vi "DMC CLI VI Analyzer.vi"() -> ()   [LabVIEW 2023]
uses:
  VIA Results Handling/Ranking Thresholds.ctl
  VI Analyzer State.ctl
  <vilib>/Wiresmith Technology/G CLI/CLI Class/CLI.lvclass
  <vilib>/addons/analyzer/_analyzerctrls.llb/VIAnAPI Ref.ctl
  <vilib>/addons/analyzer/_analyzerctrls.llb/VIAnCtl Results.ctl
  <vilib>/addons/analyzer/_analyzerctrls.llb/VIAnCtl ResultsData (index).ctl
  <vilib>/addons/analyzer/_analyzerctrls.llb/VIAnCtl ResultStatus.ctl
  <vilib>/addons/analyzer/_vianresshared.llb/VIAnRes Parsed Results Data (by VI).ctl
  <vilib>/addons/analyzer/_vianresshared.llb/VIAnRes Parsed Results Data (by Test).ctl
  <vilib>/addons/analyzer/_analyzerctrls.llb/VIAnCtl Test Config Data.ctl
  <vilib>/addons/analyzer/_analyzerctrls.llb/VIAnCtl TestRanking.ctl
  <vilib>/addons/analyzer/_analyzerctrls.llb/VIAnCtl Config Control Value.ctl
  <vilib>/Wiresmith Technology/G CLI/Argument Parser/Option Set Class/Option Set.lvclass
  <vilib>/Wiresmith Technology/G CLI/Argument Parser/Option Class/Option Configuration.ctl
  <vilib>/Wiresmith Technology/G CLI/Argument Parser/Option Class/Argument Type.ctl
  07fc47aa-534d-44f0-8168-3e6c46d68514.vi
  <vilib>/addons/analyzer/NI_VIAnalyzerTKVIs.lvlib
  <vilib>/Wiresmith Technology/G CLI/Argument Parser/Option Class/Option.lvclass
  VIA Results Handling/VIA Results Handling.lvlib
panel:
  out "File Paths":path[](array[path])
  out "Custom Parameters":string[](array[string])
  out "Ranking Thresholds":T1={"High"=100.0, "Normal"=90.0, "Low"=80.0}
  out "Per VI Threshold":bool
  out "RSL Report":bool
  out "HTML Report":bool
  out "Excluded Folders":string[](array[string])
  out "Included Folders":string[](array[string])
  in  "Show Results Window?":bool
  out "Results":string
  out "VI in Analysis":string
  out "% Complete":dbl(slide) scale=0.0..100.0
  out "# VIs to Analyze":i32
  out "Report Path":path
  out "Viancfg Path":path
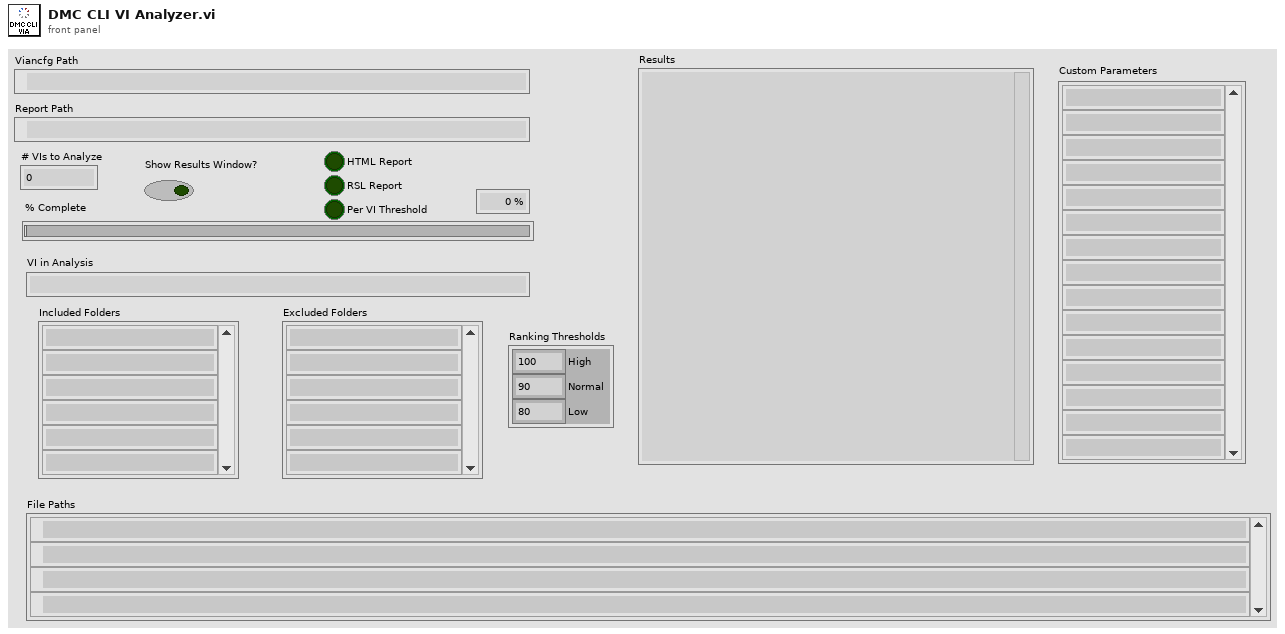
[diagram p1: front panel]
types:
  T1 = typedef "VIA Results Handling.lvlib/Ranking Thresholds.ctl" = cluster{"High":dbl, "Normal":dbl, "Low":dbl}
  T2 = typedef "VIAnAPI Ref.ctl" = refnum<k1>
  T3 = typedef "VIAnCtl Results.ctl" = cluster{"Test Name":string, "Results Data":T4[], "Status":T5, "Exceed Max Fails?":bool}
  T4 = typedef "VIAnCtl ResultsData (index).ctl" = cluster{"Result Message":string, "Ref Index":i32}
  T5 = typedef "VIAnCtl ResultStatus.ctl" = enum16{"Pass", "Fail", "Skipped", "VI not loadable", "Test not loadable", "Test not runnable", "Test error out"}
  T6 = typedef "VIAnRes Parsed Results Data (by VI).ctl" = cluster{"VI Path":path, "Pass":cluster{"row":i32, "column":i32}[], "Fail":cluster{"row":i32, "column":i32}[], "Skipped":cluster{"row":i32, "column":i32}[], "VI not loadable":cluster{"row":i32, "column":i32}[], "Test not loadable":cluster{"row":i32, "column":i32}[], "Test not runnable":cluster{"row":i32, "column":i32}[], "Test error out":cluster{"row":i32, "column":i32}[]}
  T7 = typedef "VIAnRes Parsed Results Data (by Test).ctl" = cluster{"Test Name":string, "Pass":cluster{"VI Path":path, "index":cluster{"row":i32, "column":i32}}[], "Fail":cluster{"VI Path":path, "index":cluster{"row":i32, "column":i32}}[], "Skipped":cluster{"VI Path":path, "index":cluster{"row":i32, "column":i32}}[]}
  T8 = typedef "VIAnCtl Test Config Data.ctl" = cluster{"Test Name":string, "Config Ref":refnum<vi>, "Ref Valid?":bool, "Test Ranking":T9, "Max Failures":u32, "Test Path":path, "Control Values":T10[], "Selected?":bool}
  T9 = typedef "VIAnCtl TestRanking.ctl" = u16
  T10 = typedef "VIAnCtl Config Control Value.ctl" = cluster{"Control Name":string, "Control Value":variant}
  T11 = cluster{"Viancfg Path":path, "Report Directory":path, "CLI":refnum<class "CLI.lvclass">, "VI Analyzer Task":T2, "Analysis Results":cluster{"Raw Results":T3[][], "Parsed Results Data (by VI)":T6[], "Parsed Results Data (by Test)":T7[], "Summary Statistics":cluster{"Passed Tests":i32, "Failed Tests":i32, "Skipped Tests":i32, "VIs not loadable":i32, "Tests not loadable":i32, "Tests not runnable":i32, "Test error out":i32, "Start Time":u32, "Total Time (s)":dbl}, "Test Config Data":T8[]}, "Option Set":refnum<class "Option Set.lvclass">, "Working Directory":path, "Ranking Thresholds":T1, "Included Folders":string[], "Excluded Folders":string[], "HTML Report":bool, "RSL Report":bool, "Per VI Threshold":bool, "Threshold Pass":bool}
  T12 = typedef "VI Analyzer State.ctl" = enum16{"Initialize", "Open viancfg", "Run viancfg", "Include Folders", "Exclude Folders", "Report Threshold", "Report HTML", "Report RSL", "Close", "Help"}
  T13 = enum16{"Viancfg Path", "Report Directory", "Included Folders", "Excluded Folders", "HTML Report", "RSL Report", "Thresholds", "Per VI Threshold"}
  T14 = typedef "Option Parser.lvlib/Option.lvclass/Option Configuration.ctl" = cluster{"Option Type":T15, "Option Labels":string[], "Key":string, "Description":string, "Required":bool, "Default Value":string}
  T15 = typedef "Option Parser.lvlib/Option.lvclass/Argument Type.ctl" = enum16{"flag", "value"}
  T16 = enum16{"open", "replace", "create", "open or create", "replace or create", "replace or create with confirmation"}
  T17 = enum16{"Viancfg Path", "Report Directory", "Included Folders", "Excluded Folders", "HTML Report", "RSL Report", "Thresholds", "Per VI Threshold"}[]
  T18 = cluster{"Raw Results":T3[][], "Parsed Results Data (by VI)":T6[], "Parsed Results Data (by Test)":T7[], "Summary Statistics":cluster{"Passed Tests":i32, "Failed Tests":i32, "Skipped Tests":i32, "VIs not loadable":i32, "Tests not loadable":i32, "Tests not runnable":i32, "Test error out":i32, "Start Time":u32, "Total Time (s)":dbl}, "Test Config Data":T8[]}
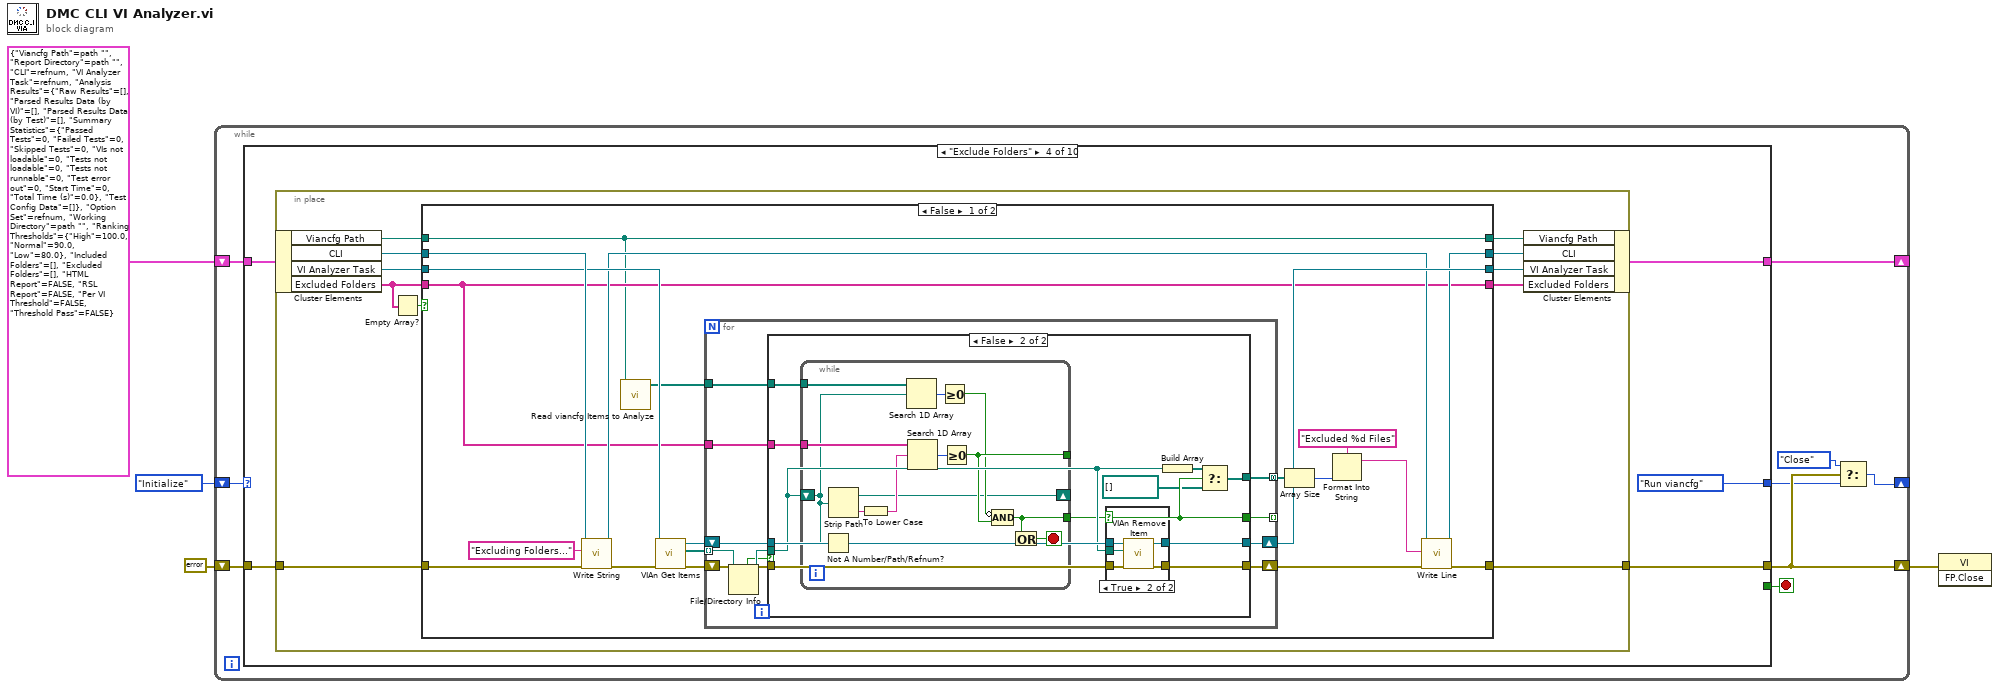
[diagram p0: block diagram]
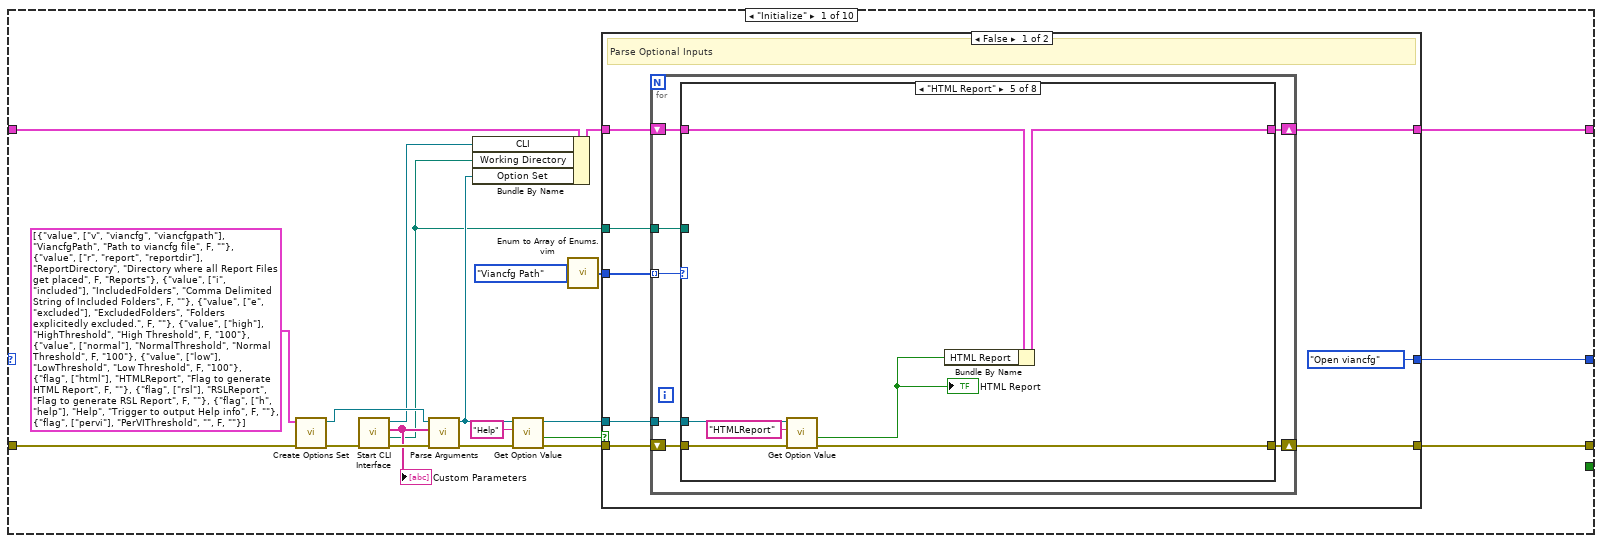
[diagram p2: hidden frame]
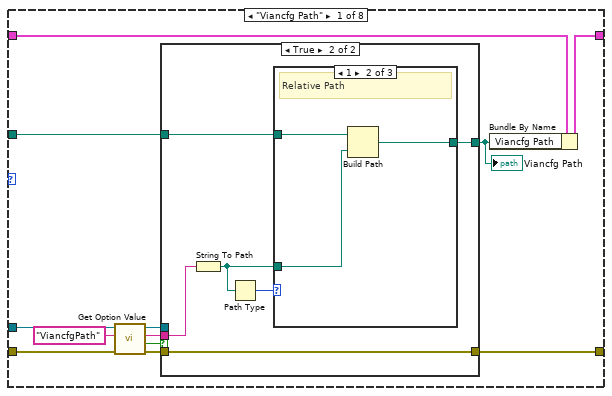
[diagram p3: hidden frame]
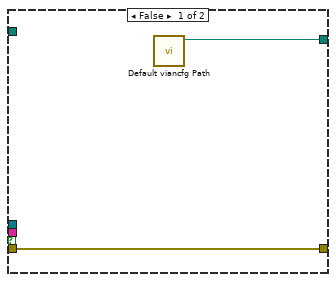
[diagram p4: hidden frame]
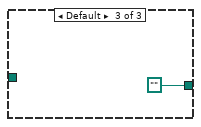
[diagram p6: hidden frame]
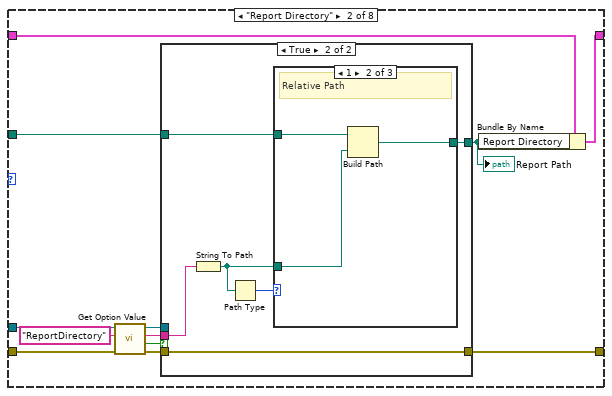
[diagram p7: hidden frame]
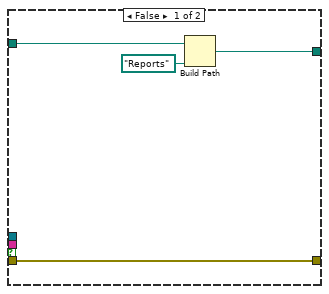
[diagram p8: hidden frame]
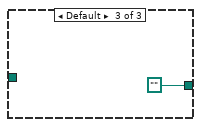
[diagram p10: hidden frame]
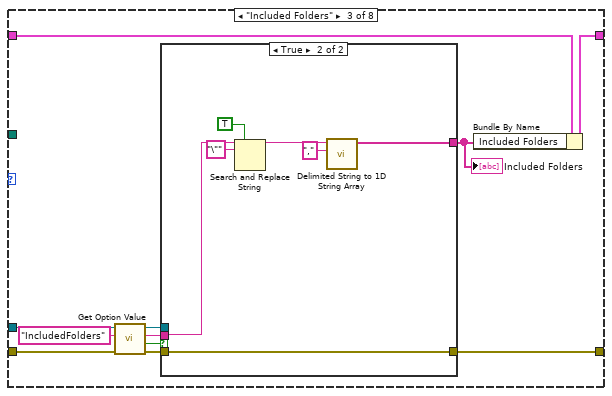
[diagram p11: hidden frame]
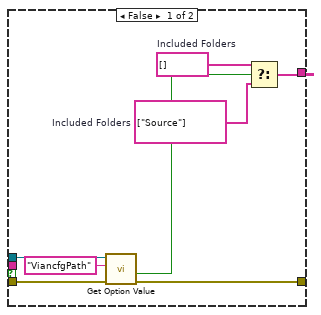
[diagram p12: hidden frame]
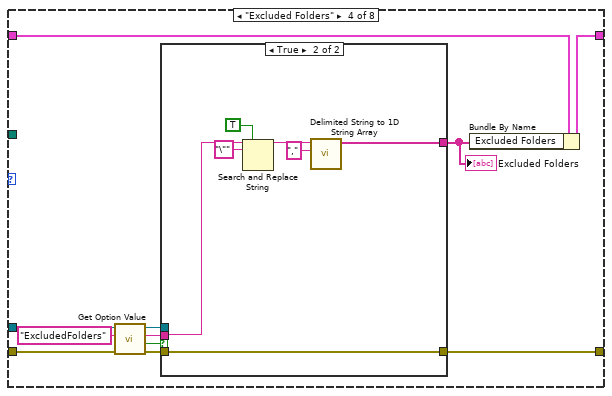
[diagram p13: hidden frame]
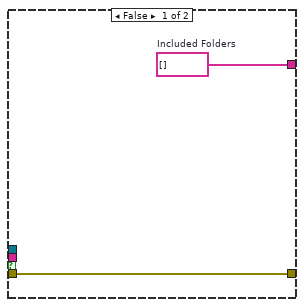
[diagram p14: hidden frame]
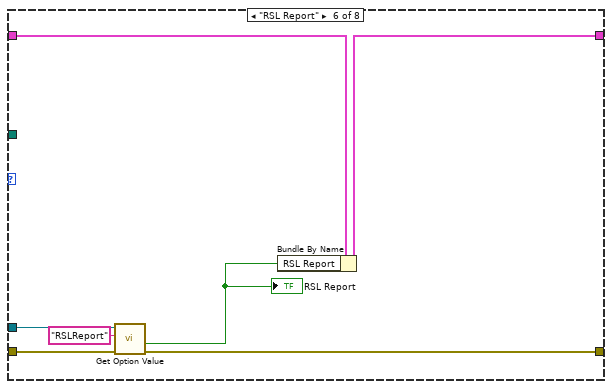
[diagram p15: hidden frame]
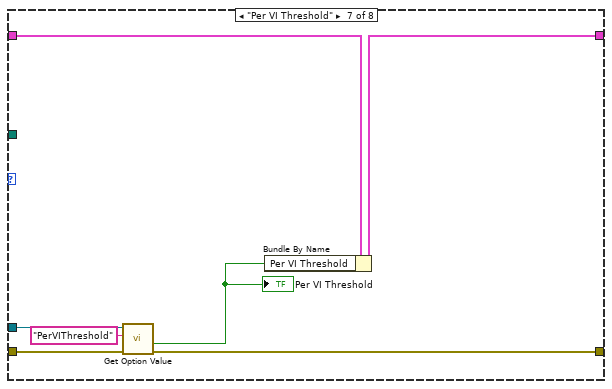
[diagram p16: hidden frame]
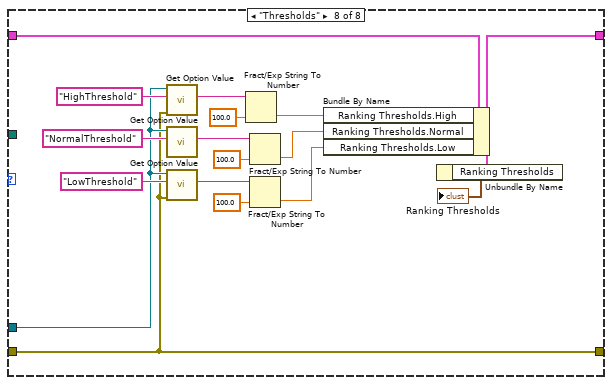
[diagram p17: hidden frame]
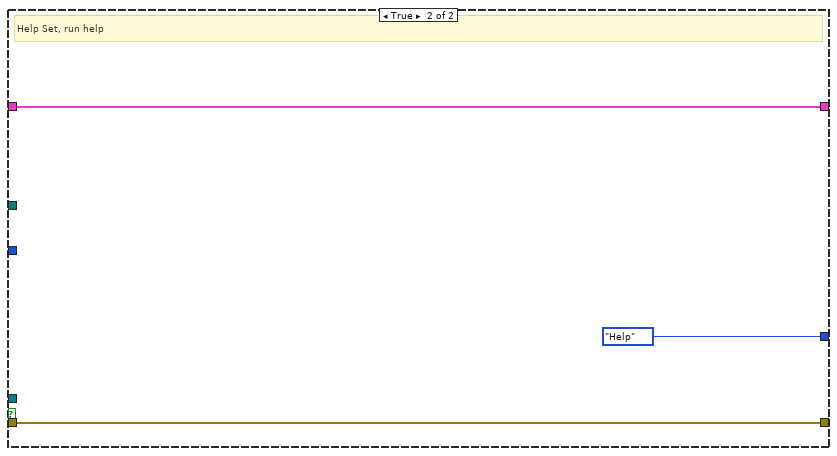
[diagram p18: hidden frame]
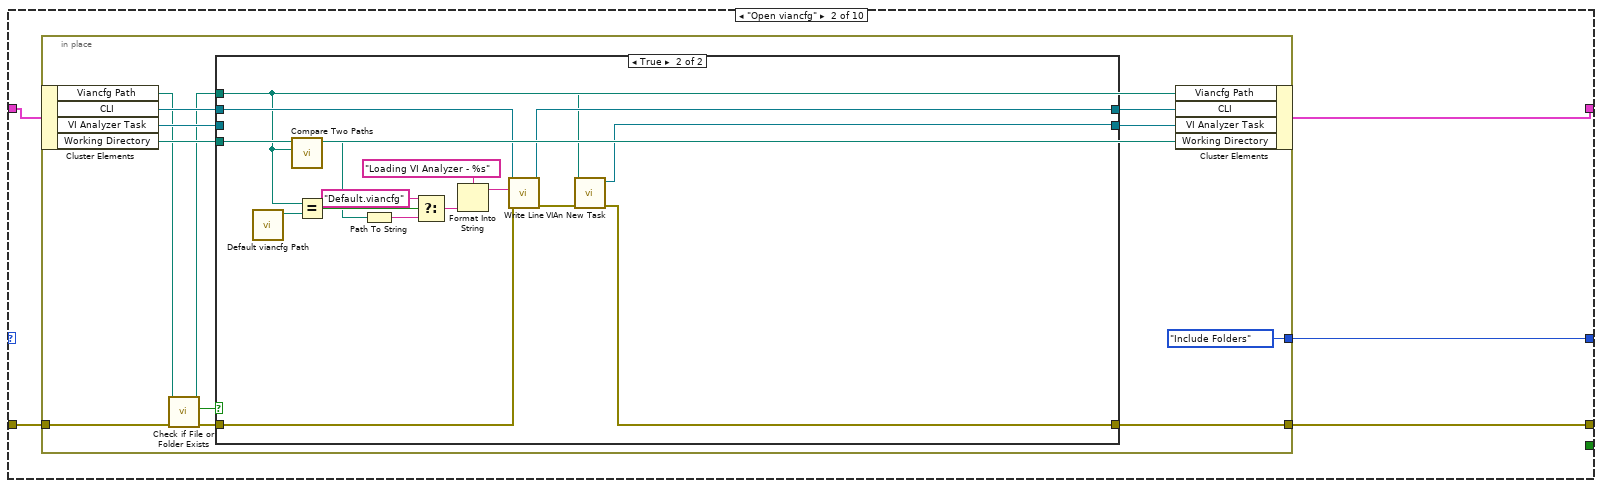
[diagram p19: hidden frame]
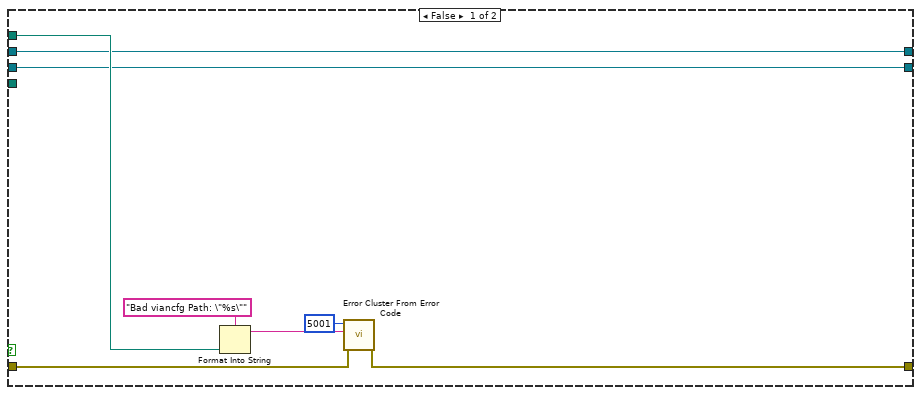
[diagram p20: hidden frame]
diagram:
  n1 = while {
    shift-right: [w6] -> _
    shift-left: VI_Analyzer_State."Initialize" -> [w13]
    shift-right: [w10] -> _
    shift-left: T11 {"Viancfg Path"=path "", "Report Directory"=path "", "CLI"=refnum, "VI Analyzer Task"=refnum, "Analysis Results"={"Raw Results"=[], "Parsed Results Data (by VI)"=[], "Parsed Results Data (by Test)"=[], "Summary Statistics"={"Passed Tests"=0, "Failed Tests"=0, "Skipped Tests"=0, "VIs not loadable"=0, "Tests not loadable"=0, "Tests not runnable"=0, "Test error out"=0, "Start Time"=0, "Total Time (s)"=0.0}, "Test Config Data"=[]}, "Option Set"=refnum, "Working Directory"=path "", "Ranking Thresholds"={"High"=100.0, "Normal"=90.0, "Low"=80.0}, "Included Folders"=[], "Excluded Folders"=[], "HTML Report"=FALSE, "RSL Report"=FALSE, "Per VI Threshold"=FALSE, "Threshold Pass"=FALSE} -> [w12]
    shift-right: [w9] -> w1
    shift-left: errorcluster {"status"=FALSE, "code"=0, "source"=""} ("error out") -> [w11]
    stop <- w5 stop-if-true
    n2 = case shown="\"Exclude Folders\"" w13 {
      tunnel: w12 -> [w34 w193 w234 w322 w438 w506 w540 w573 w619 w621]
      tunnel: w11 -> [w29 w190 w231 w319 w436 w509 w543 w576 w618 w623]
      tunnel: [w14 w192 w233 w321 w437 w510 w544 w577 w619 w620] -> w10
      tunnel: [w18 w191 w232 w320 w435 w508 w542 w575 w615 w622] -> w9
      tunnel: [w33 w189 VI_Analyzer_State."Exclude Folders" VI_Analyzer_State."Run viancfg" w434 w507 w541 w574 VI_Analyzer_State."Close" VI_Analyzer_State."Close"] -> w7
      tunnel: [_ _ _ _ _ _ _ _ TRUE _] -> w5
      frame "Initialize" {
        n3 = call <vilib>:"Create Options Set.vi"("error in (no error)"=w29, "Options"=T14[] [{"Option Type"=enum."value", "Option Labels"=["v", "viancfg", "viancfgpath"], "Key"="ViancfgPath", "Description"="Path to viancfg file", "Required"=FALSE, "Default Value"=""}, {"Option Type"=enum."value", "Option Labels"=["r", "report", "reportdir"], "Key"="ReportDirectory", "Description"="Directory where all Report Files get placed", "Required"=FALSE, "Default Value"="Reports"}, {"Option Type"=enum."value", "Option Labels"=["i", "included"], "Key"="IncludedFolders", "Description"="Comma Delimited String of Included Folders", "Required"=FALSE, "Default Value"=""}, {"Option Type"=enum."value", "Option Labels"=["e", "excluded"], "Key"="ExcludedFolders", "Description"="Folders explicitedly excluded.", "Required"=FALSE, "Default Value"=""}, {"Option Type"=enum."value", "Option Labels"=["high"], "Key"="HighThreshold", "Description"="High Threshold", "Required"=FALSE, "Default Value"="100"}, {"Option Type"=enum."value", "Option Labels"=["normal"], "Key"="NormalThreshold", "Description"="Normal Threshold", "Required"=FALSE, "Default Value"="100"}, {"Option Type"=enum."value", "Option Labels"=["low"], "Key"="LowThreshold", "Description"="Low Threshold", "Required"=FALSE, "Default Value"="100"}, {"Option Type"=enum."flag", "Option Labels"=["html"], "Key"="HTMLReport", "Description"="Flag to generate HTML Report", "Required"=FALSE, "Default Value"=""}, {"Option Type"=enum."flag", "Option Labels"=["rsl"], "Key"="RSLReport", "Description"="Flag to generate RSL Report", "Required"=FALSE, "Default Value"=""}, {"Option Type"=enum."flag", "Option Labels"=["h", "help"], "Key"="Help", "Description"="Trigger to output Help info", "Required"=FALSE, "Default Value"=""}, {"Option Type"=enum."flag", "Option Labels"=["pervi"], "Key"="PerVIThreshold", "Description"="", "Required"=FALSE, "Default Value"=""}]) -> ("error out"=w30:errorcluster, "Option Set out"=w28:refnum<class "Option Set.lvclass">)  [unwired: 8 in]
        n4 = call <vilib>:"Start CLI Interface.vi"("error in (no error)"=w30) -> ("error out"=w32:errorcluster, "Working Directory"=w15:path, "Custom Parameters"=w27:string[], "CLI out"=w23:refnum<class "CLI.lvclass">)  [unwired: 7 in]
        "Custom Parameters" <- w27
        n5 = call <vilib>:"Parse Arguments.vi"("error in (no error)"=w32, "Arguments"=w27, "Option Set in"=w28) -> ("error out"=w25:errorcluster, "Option Set out"=w22:refnum<class "Option Set.lvclass">)  [unwired: 5 in, 2 out]
        n6 = Bundle By Name(cluster=w34, "CLI"=w23, "Working Directory"=w15, "Option Set"=w22) -> (w24:T11)
        n7 = call <vilib>:"Get Option Value.vi"("error in (no error)"=w25, "Option Key"="Help", "Option Set in"=w22) -> ("error out"=w20:errorcluster, "Set"=w21:bool, "Option Set out"=w19:refnum<class "Option Set.lvclass">)  [unwired: 5 in, 1 out]
        n8 = call "Enum to Array of Enums.vim"("enum"=T13."Viancfg Path") -> ("array of enums"=w16:T17)
        n9 = case shown="False" w21 {
          tunnel: [w38 w187] -> w14
          tunnel: [VI_Analyzer_State."Open viancfg" VI_Analyzer_State."Help"] -> w33
          tunnel: w24 -> [w40 w187]
          tunnel: w20 -> [w41 w186]
          tunnel: w19 -> [w42 _]
          tunnel: [w36 w186] -> w18
          tunnel: w16 -> [w39 _]
          tunnel: w15 -> [w37 _]
          frame False {
            # "Parse Optional Inputs"
            n10 = for {
              tunnel: w42 -> [w49]
              shift-right: [w46] -> w38
              shift-left: w40 -> [w45]
              tunnel: w39 -> [w47] mode=indexing
              tunnel: w37 -> [w44]
              shift-right: [w43] -> w36
              shift-left: w41 -> [w48]
              n11 = case shown="\"HTML Report\"" w47 {
                tunnel: w49 -> [w61 w86 w112 w138 w154 w161 w168 w178]
                tunnel: w48 -> [w60 w85 w111 w137 w153 w160 w167 w177]
                tunnel: [w52 w77 w103 w129 w149 w156 w163 w170] -> w46
                tunnel: w45 -> [w54 w79 w105 w131 w151 w158 w165 w184]
                tunnel: w44 -> [w51 w76 _ _ _ _ _ _]
                tunnel: [w53 w78 w104 w130 w150 w157 w164 w177] -> w43
                frame "Viancfg Path" {
                  n12 = call <vilib>:"Get Option Value.vi"("error in (no error)"=w60, "Option Key"="ViancfgPath", "Option Set in"=w61) -> ("error out"=w58:errorcluster, "Set"=w57:bool, "Value"=w55:string, "Option Set out"=w56:refnum<class "Option Set.lvclass">)  [unwired: 5 in]
                  n13 = case shown="True" w57 {
                    tunnel: w58 -> [w63 w68]
                    tunnel: w56 -> [_ _]
                    tunnel: w55 -> [_ w69]
                    tunnel: [w63 w68] -> w53
                    tunnel: [w62 w65] -> w50
                    tunnel: w51 -> [_ w64]
                    frame False {
                      n14 = call "Default viancfg Path.vi"() -> ("Default.viancfg Path"=w62:path)  [unwired: 11 in]
                    }
                    frame True {
                      n15 = String To Path(string=w69) -> (path=w66:path)
                      n16 = Path Type(1:w66) -> (0:w67:i16)
                      n17 = case shown="1" w67 {
                        tunnel: w66 -> [w70 w72 _]
                        tunnel: [w70 w71 path ""] -> w65
                        tunnel: w64 -> [_ w73 _]
                        frame 0 {
                          # "Absolute Path"
                        }
                        frame 1 {
                          # "Relative Path"
                          n18 = Build Path(base path=w73, name or relative path=w72) -> (appended path=w71:path)
                        }
                        frame Default {
                        }
                      }
                    }
                  }
                  "Viancfg Path" <- w50
                  n19 = Bundle By Name(cluster=w54, "Viancfg Path"=w50) -> (w52:T11)
                }
                frame "Report Directory" {
                  n20 = call <vilib>:"Get Option Value.vi"("error in (no error)"=w85, "Option Key"="ReportDirectory", "Option Set in"=w86) -> ("error out"=w83:errorcluster, "Set"=w82:bool, "Value"=w80:string, "Option Set out"=w81:refnum<class "Option Set.lvclass">)  [unwired: 5 in]
                  n21 = case shown="True" w82 {
                    tunnel: w83 -> [w89 w95]
                    tunnel: w81 -> [_ _]
                    tunnel: w80 -> [_ w96]
                    tunnel: [w89 w95] -> w78
                    tunnel: [w88 w92] -> w75
                    tunnel: w76 -> [w87 w91]
                    frame False {
                      n22 = Build Path(base path=w87, name or relative path=path "Reports") -> (appended path=w88:path)
                    }
                    frame True {
                      n23 = String To Path(string=w96) -> (path=w93:path)
                      n24 = Path Type(1:w93) -> (0:w94:i16)
                      n25 = case shown="1" w94 {
                        tunnel: w93 -> [w97 w99 _]
                        tunnel: [w97 w98 path ""] -> w92
                        tunnel: w91 -> [_ w100 _]
                        frame 0 {
                          # "Absolute Path"
                        }
                        frame 1 {
                          # "Relative Path"
                          n26 = Build Path(base path=w100, name or relative path=w99) -> (appended path=w98:path)
                        }
                        frame Default {
                        }
                      }
                    }
                  }
                  "Report Path" <- w75
                  n27 = Bundle By Name(cluster=w79, "Report Directory"=w75) -> (w77:T11)
                }
                frame "Included Folders" {
                  n28 = call <vilib>:"Get Option Value.vi"("error in (no error)"=w111, "Option Key"="IncludedFolders", "Option Set in"=w112) -> ("error out"=w109:errorcluster, "Set"=w108:bool, "Value"=w106:string, "Option Set out"=w107:refnum<class "Option Set.lvclass">)  [unwired: 5 in]
                  n29 = case shown="True" w108 {
                    tunnel: w109 -> [w118 w127]
                    tunnel: w107 -> [w119 _]
                    tunnel: w106 -> [_ w122]
                    tunnel: [w117 w127] -> w104
                    tunnel: [w113 w126] -> w102
                    frame False {
                      w114 = string[] ["Source"]  # Included Folders
                      w115 = string[] []  # Included Folders
                      n30 = call <vilib>:"Get Option Value.vi"("error in (no error)"=w118, "Option Key"="ViancfgPath", "Option Set in"=w119) -> ("error out"=w117:errorcluster, "Set"=w116:bool)  [unwired: 5 in, 2 out]
                      n31 = Select(t=w115, s=w116, f=w114) -> (s? t:f=w113:string[])
                    }
                    frame True {
                      n32 = Search and Replace String(replace all?=TRUE ("replace all? (F)"), input string=w122, search string="\"") -> (result string=w123:string)  [unwired: 5 in, 3 out]
                      n33 = call <vilib>:"Delimited String to 1D String Array.vi"("delimiter"=",", "delimited string"=w123) -> ("string array"=w126:string[])  [unwired: 9 in]
                    }
                  }
                  "Included Folders" <- w102
                  n34 = Bundle By Name(cluster=w105, "Included Folders"=w102) -> (w103:T11)
                }
                frame "Excluded Folders" {
                  n35 = call <vilib>:"Get Option Value.vi"("error in (no error)"=w137, "Option Key"="ExcludedFolders", "Option Set in"=w138) -> ("error out"=w135:errorcluster, "Set"=w134:bool, "Value"=w132:string, "Option Set out"=w133:refnum<class "Option Set.lvclass">)  [unwired: 5 in]
                  n36 = case shown="True" w134 {
                    tunnel: w135 -> [w140 w147]
                    tunnel: w133 -> [_ _]
                    tunnel: w132 -> [_ w141]
                    tunnel: [w140 w147] -> w130
                    tunnel: [w139 w146] -> w128
                    frame False {
                      w139 = string[] []  # Included Folders
                    }
                    frame True {
                      n37 = Search and Replace String(replace all?=TRUE ("replace all? (F)"), input string=w141, search string="\"") -> (result string=w142:string)  [unwired: 5 in, 3 out]
                      n38 = call <vilib>:"Delimited String to 1D String Array.vi"("delimiter"=",", "delimited string"=w142) -> ("string array"=w146:string[])  [unwired: 9 in]
                    }
                  }
                  "Excluded Folders" <- w128
                  n39 = Bundle By Name(cluster=w131, "Excluded Folders"=w128) -> (w129:T11)
                }
                frame "HTML Report" {
                  n40 = call <vilib>:"Get Option Value.vi"("error in (no error)"=w153, "Option Key"="HTMLReport", "Option Set in"=w154) -> ("error out"=w150:errorcluster, "Set"=w148:bool)  [unwired: 5 in, 2 out]
                  "HTML Report" <- w148
                  n41 = Bundle By Name(cluster=w151, "HTML Report"=w148) -> (w149:T11)
                }
                frame "RSL Report" {
                  n42 = call <vilib>:"Get Option Value.vi"("error in (no error)"=w160, "Option Key"="RSLReport", "Option Set in"=w161) -> ("error out"=w157:errorcluster, "Set"=w155:bool)  [unwired: 5 in, 2 out]
                  "RSL Report" <- w155
                  n43 = Bundle By Name(cluster=w158, "RSL Report"=w155) -> (w156:T11)
                }
                frame "Per VI Threshold" {
                  n44 = call <vilib>:"Get Option Value.vi"("error in (no error)"=w167, "Option Key"="PerVIThreshold", "Option Set in"=w168) -> ("error out"=w164:errorcluster, "Set"=w162:bool)  [unwired: 5 in, 2 out]
                  "Per VI Threshold" <- w162
                  n45 = Bundle By Name(cluster=w165, "Per VI Threshold"=w162) -> (w163:T11)
                }
                frame "Thresholds" {
                  n46 = call <vilib>:"Get Option Value.vi"("error in (no error)"=w177, "Option Key"="HighThreshold", "Option Set in"=w178) -> ("Value"=w183:string)  [unwired: 5 in, 3 out]
                  n47 = call <vilib>:"Get Option Value.vi"("Option Key"="NormalThreshold", "Option Set in"=w178) -> ("Value"=w175:string)  [unwired: 6 in, 3 out]
                  n48 = call <vilib>:"Get Option Value.vi"("error in (no error)"=w177, "Option Key"="LowThreshold", "Option Set in"=w178) -> ("Value"=w172:string)  [unwired: 5 in, 3 out]
                  n49 = Fract/Exp String To Number(string=w183, default (0 dbl)=100.0 ("default (0 DBL)")) -> (number=w182:dbl)  [unwired: 2 in, 1 out]
                  n50 = Fract/Exp String To Number(string=w175, default (0 dbl)=100.0 ("default (0 DBL)")) -> (number=w174:dbl)  [unwired: 2 in, 1 out]
                  n51 = Fract/Exp String To Number(string=w172, default (0 dbl)=100.0 ("default (0 DBL)")) -> (number=w171:dbl)  [unwired: 2 in, 1 out]
                  n52 = Bundle By Name(cluster=w184, "Ranking Thresholds.High"=w182, "Ranking Thresholds.Normal"=w174, "Ranking Thresholds.Low"=w171) -> (w170:T11)
                  n53 = Unbundle By Name(w170) -> ("Ranking Thresholds"=→"Ranking Thresholds":T1)
                }
              }
            }
          }
          frame True {
            # "Help Set, run help"
          }
        }
      }
      frame "Open viancfg" {
        n54 = in-place {
          in-place-border: [w203] -> w191
          in-place-border: w190 -> [w194]
          in-place-border: [VI_Analyzer_State."Include Folders"] -> w189
          n55 = in-place-cluster #1(w193) -> ("Viancfg Path"=w198:path, "CLI"=w205:refnum<class "CLI.lvclass">, "VI Analyzer Task"=w202:T2, "Working Directory"=w199:path)
          n56 = call <vilib>:"Check if File or Folder Exists.vi"("error in (no error)"=w194, "path"=w198) -> ("error out"=w195:errorcluster, "file or folder exists?"=w196:bool, "dup path"=w197:path)  [unwired: 7 in]
          n57 = case shown="True" w196 {
            tunnel: w205 -> [w211 w228]
            tunnel: [w211 w225] -> w204
            tunnel: [w208 w224] -> w203
            tunnel: w195 -> [w209 w227]
            tunnel: w197 -> [w212 w219]
            tunnel: w202 -> [w206 _]
            tunnel: [w206 w226] -> w200
            tunnel: w199 -> [_ w223]
            frame False {
              n58 = Format Into String(format string="Bad viancfg Path: \"%s\"", w212) -> (resulting string=w210:string)  [unwired: 2 in, 1 out]
              n59 = call <vilib>:"Error Cluster From Error Code.vi"("error in (no error)"=w209, "error message (\"\")"=w210, "error code (0)"=5001) -> ("error out"=w208:errorcluster)  [unwired: 6 in]
            }
            frame True {
              n60 = call "Default viancfg Path.vi"() -> ("Default.viancfg Path"=w220:path)  [unwired: 11 in]
              n61 = call <vilib>:"Compare Two Paths.vi"("Path 2"=w219, "Path 1"=w223) -> ("Relative Path from 1 to 2"=w215:path)  [unwired: 6 in, 3 out]
              n62 = Equal?(x=w219, y=w220) -> (x = y?=w218:bool)
              n63 = Path To String(path=w215) -> (string=w214:string)
              n64 = Select(t="Default.viancfg", s=w218, f=w214) -> (s? t:f=w216:string)
              n65 = Format Into String(format string="Loading VI Analyzer - %s" ("Text to Write"), w216) -> (resulting string=w221:string)  [unwired: 2 in, 1 out]
              n66 = call <vilib>:"Write Line.vi"("error in (no error)"=w227, "Text to Write"=w221, "CLI in"=w228) -> ("error out"=w229:errorcluster, "CLI out"=w225:refnum<class "CLI.lvclass">)  [unwired: 7 in]
              n67 = call <vilib>:"VIAn New Task.vi"("error in (no error)"=w229, "Path to Configuration File"=w219) -> ("error out"=w224:errorcluster, "VI Analyzer Task"=w226:T2)  [unwired: 8 in]
            }
          }
          n68 = in-place-cluster #1("Viancfg Path"=w197, "CLI"=w204, "VI Analyzer Task"=w200, "Working Directory"=w199) -> (w192:T11)
        }
      }
      frame "Include Folders" {
        n69 = in-place {
          in-place-border: [w243] -> w232
          in-place-border: w231 -> [w242]
          n70 = in-place-cluster #2(w234) -> ("Working Directory"=w236:path, "CLI"=w245:refnum<class "CLI.lvclass">, "VI Analyzer Task"=w240:T2, "Included Folders"=w239:string[])
          n71 = Empty Array?(array=w239) -> (empty?=w237:bool)
          n72 = case shown="False" w237 {
            tunnel: w245 -> [w271 w317]
            tunnel: [w252 w317] -> w244
            tunnel: [w254 w314] -> w243
            tunnel: w242 -> [w250 w314]
            tunnel: [w259 w316] -> w241
            tunnel: w240 -> [w268 w316]
            tunnel: w239 -> [w262 w315]
            tunnel: [w262 w315] -> w238
            tunnel: w236 -> [w248 w313]
            tunnel: [w248 w313] -> w235
            frame False {
              n73 = call <vilib>:"Write String.vi"("error in (no error)"=w250, "Text to Write"="Setting Included Folders...", "CLI in"=w271) -> ("error out"=w270:errorcluster, "CLI out"=w253:refnum<class "CLI.lvclass">)  [unwired: 7 in]
              n74 = call <vilib>:"VIAn Get Items.vi"("error in (no error)"=w270, "VI Analyzer Task in"=w268) -> ("error out"=w267:errorcluster, "Items"=w265:path[], "VI Analyzer Task out"=w266:T2)  [unwired: 7 in]
              n75 = for {
                shift-right: [w310] -> w263
                shift-left: w266 -> [w312]
                shift-right: [w309] -> w264
                shift-left: w267 -> [w311]
                tunnel: w265 -> [w308] mode=indexing
                n76 = call <vilib>:"VIAn Remove Item.vi"("error in (no error)"=w311, "Item to Remove"=w308, "VI Analyzer Task in"=w312) -> ("error out"=w309:errorcluster, "VI Analyzer Task out"=w310:T2)  [unwired: 7 in]
              }
              n77 = call <vilib>:"Recursive File List.vi"("pattern"="*.vi", "error in (no error)"=w250, "Folder Path"=w248) -> ("error out"=w249:errorcluster, "All Files in Dir"=w247:path[])  [unwired: 4 in, 3 out]
              n78 = To Lower Case(string=w262) -> (all lower case string=w261:string[])
              n79 = Merge Errors(w264, w249) -> (w260:errorcluster)
              n80 = for {
                shift-right: [w281] -> w259
                shift-left: w263 -> [w282]
                shift-right: [w280] -> w255
                shift-left: w260 -> [w273]
                tunnel: w247 -> [w274] mode=indexing
                tunnel: w261 -> [w279]
                tunnel: [w278] -> w257 mode=indexing if=w277
                n81 = call <vilib>:"Check if File or Folder Exists.vi"("error in (no error)"=w273, "path"=w274) -> ("error out"=w272:errorcluster, "file or folder exists?"=w276:bool, "dup path"=w275:path)  [unwired: 7 in]
                n82 = case shown="True" w276 {
                  tunnel: w282 -> [w284 w291]
                  tunnel: w272 -> [w283 w290]
                  tunnel: [w284 w289] -> w281
                  tunnel: [w283 w288] -> w280
                  tunnel: w275 -> [_ w286]
                  tunnel: w279 -> [_ w287]
                  tunnel: [_ w286] -> w278
                  tunnel: [_ w285] -> w277
                  frame False {
                  }
                  frame True {
                    n83 = while {
                      tunnel: w287 -> [w306]
                      tunnel: [w299] -> w285
                      shift-right: [w303] -> _
                      shift-left: w286 -> [w302]
                      stop <- w301 stop-if-true
                      n84 = Not A Number/Path/Refnum?(number/path/refnum=w302) -> (NaN/Path/Refnum?=w300:bool)
                      n85 = Strip Path(path=w302) -> (stripped path=w303:path, name=w307:string)
                      n86 = To Lower Case(string=w307) -> (all lower case string=w305:string)
                      n87 = Search 1D Array(1D array=w306, element=w305) -> (index of element=w304:i32)  [unwired: 1 in]
                      n88 = Greater Or Equal To 0?(x=w304) -> (x >= 0?=w299:bool)
                      n89 = Or(x=w299, y=w300) -> (x .or. y?=w301:bool)
                    }
                    n90 = case shown="True" w285 {
                      tunnel: w291 -> [w293 w298]
                      tunnel: w290 -> [w292 w297]
                      tunnel: [w293 w296] -> w289
                      tunnel: [w292 w295] -> w288
                      tunnel: w286 -> [_ w294]
                      frame False {
                      }
                      frame True {
                        n91 = call <vilib>:"VIAn Add Item.vi"("error in (no error)"=w297, "Item to Add"=w294, "VI Analyzer Task in"=w298) -> ("error out"=w295:errorcluster, "VI Analyzer Task out"=w296:T2)  [unwired: 7 in]
                      }
                    }
                  }
                }
              }
              n92 = Array Size(array=w257) -> (size(s)=w258:i32)
              n93 = Format Into String(format string="Included %d files", w258) -> (resulting string=w251:string)  [unwired: 2 in, 1 out]
              n94 = call <vilib>:"Write Line.vi"("error in (no error)"=w255, "Text to Write"=w251, "CLI in"=w253) -> ("error out"=w254:errorcluster, "CLI out"=w252:refnum<class "CLI.lvclass">)  [unwired: 7 in]
            }
            frame True {
            }
          }
          n95 = in-place-cluster #2("Working Directory"=w235, "CLI"=w244, "VI Analyzer Task"=w241, "Included Folders"=w238) -> (w233:T11)
        }
      }
      frame "Exclude Folders" {
        n96 = in-place {
          in-place-border: [w331] -> w320
          in-place-border: w319 -> [w330]
          n97 = in-place-cluster #3(w322) -> ("Viancfg Path"=w324:path, "CLI"=w333:refnum<class "CLI.lvclass">, "VI Analyzer Task"=w328:T2, "Excluded Folders"=w327:string[])
          n98 = Empty Array?(array=w327) -> (empty?=w325:bool)
          n99 = case shown="False" w325 {
            tunnel: w333 -> [w353 w433]
            tunnel: [w338 w433] -> w332
            tunnel: [w340 w430] -> w331
            tunnel: w330 -> [w351 w430]
            tunnel: [w342 w432] -> w329
            tunnel: w328 -> [w343 w432]
            tunnel: w327 -> [w336 w431]
            tunnel: [w336 w431] -> w326
            tunnel: w324 -> [w335 w429]
            tunnel: [w335 w429] -> w323
            frame False {
              n100 = call <vilib>:"Write String.vi"("error in (no error)"=w351, "Text to Write"="Excluding Folders...", "CLI in"=w353) -> ("error out"=w344:errorcluster, "CLI out"=w339:refnum<class "CLI.lvclass">)  [unwired: 7 in]
              n101 = call "Read viancfg Items to Analyze.vi"("viancfg Path"=w335) -> ("Removed Paths"=w334:path[])  [unwired: 8 in, 2 out]
              n102 = call <vilib>:"VIAn Get Items.vi"("error in (no error)"=w344, "VI Analyzer Task in"=w343) -> ("error out"=w350:errorcluster, "Items"=w348:path[], "VI Analyzer Task out"=w349:T2)  [unwired: 7 in]
              n103 = for {
                tunnel: w348 -> [w357] mode=indexing
                tunnel: w336 -> [w364]
                shift-right: [w361] -> w342
                shift-left: w349 -> [w363]
                shift-right: [w362] -> w341
                shift-left: w350 -> [w354]
                tunnel: w334 -> [w360]
                tunnel: [w359] -> _ mode=indexing
                tunnel: [w358] -> w346 mode=concatenating
                n104 = File/Directory Info(path=w357) -> (path out=w356:path, directory=w355:bool)  [unwired: 1 in, 5 out]
                n105 = case shown="False" w355 {
                  tunnel: w364 -> [w375 w408]
                  tunnel: w363 -> [w374 w407]
                  tunnel: w354 -> [w373 w403]
                  tunnel: [w372 w406] -> w362
                  tunnel: [w370 w405] -> w361
                  tunnel: w360 -> [w369 w404]
                  tunnel: [w366 w400] -> w359
                  tunnel: w356 -> [w367 w402]
                  tunnel: [w365 w399] -> w358
                  frame True {
                    n106 = call <vilib>:"Recursive File List.vi"("error in (no error)"=w373, "Folder Path"=w367) -> ("error out"=w371:errorcluster, "All Folders"=w376:path[])  [unwired: 5 in, 3 out]
                    n107 = for {
                      tunnel: w376 -> [w378] mode=indexing
                      tunnel: w375 -> [w389]
                      shift-right: [w385] -> w370
                      shift-left: w374 -> [w386]
                      shift-right: [w384] -> w372
                      shift-left: w371 -> [w383]
                      tunnel: w369 -> [w381]
                      tunnel: [w377] -> w368 mode=indexing
                      tunnel: [w378] -> w365 mode=indexing if=w377
                      n108 = Strip Path(path=w378) -> (name=w390:string)  [unwired: 1 out]
                      n109 = To Lower Case(string=w390) -> (all lower case string=w388:string)
                      n110 = Search 1D Array(1D array=w381, element=w378) -> (index of element=w380:i32)  [unwired: 1 in]
                      n111 = Search 1D Array(1D array=w389, element=w388) -> (index of element=w387:i32)  [unwired: 1 in]
                      n112 = Greater Or Equal To 0?(x=w380) -> (x >= 0?=w379:bool)
                      n113 = Greater Or Equal To 0?(x=w387) -> (x >= 0?=w382:bool)
                      n114 = Compound Arithmetic op=AND(invert w379, w382) -> (w377:bool)
                      n115 = case shown="True" w377 {
                        tunnel: w386 -> [w392 w397]
                        tunnel: [w392 w396] -> w385
                        tunnel: w378 -> [_ w393]
                        tunnel: [w391 w395] -> w384
                        tunnel: w383 -> [w391 w394]
                        frame False {
                        }
                        frame True {
                          n116 = call <vilib>:"VIAn Remove Item.vi"("error in (no error)"=w394, "Item to Remove"=w393, "VI Analyzer Task in"=w397) -> ("error out"=w395:errorcluster, "VI Analyzer Task out"=w396:T2)  [unwired: 7 in]
                        }
                      }
                    }
                    n117 = Or Array Elements(Boolean array=w368) -> (logical OR=w366:bool)
                  }
                  frame False {
                    n118 = while {
                      tunnel: w408 -> [w420]
                      tunnel: [w417] -> _
                      tunnel: w404 -> [w416]
                      tunnel: [w413] -> w400
                      shift-right: [w412] -> _
                      shift-left: w402 -> [w411]
                      stop <- w410 stop-if-true
                      n119 = Not A Number/Path/Refnum?(number/path/refnum=w411) -> (NaN/Path/Refnum?=w409:bool)
                      n120 = Strip Path(path=w411) -> (stripped path=w412:path, name=w421:string)
                      n121 = To Lower Case(string=w421) -> (all lower case string=w419:string)
                      n122 = Search 1D Array(1D array=w416, element=w411) -> (index of element=w415:i32)  [unwired: 1 in]
                      n123 = Search 1D Array(1D array=w420, element=w419) -> (index of element=w418:i32)  [unwired: 1 in]
                      n124 = Greater Or Equal To 0?(x=w415) -> (x >= 0?=w414:bool)
                      n125 = Greater Or Equal To 0?(x=w418) -> (x >= 0?=w417:bool)
                      n126 = Compound Arithmetic op=AND(invert w414, w417) -> (w413:bool)
                      n127 = Or(x=w413, y=w409) -> (x .or. y?=w410:bool)
                    }
                    n128 = case shown="True" w400 {
                      tunnel: w407 -> [w423 w428]
                      tunnel: [w423 w427] -> w405
                      tunnel: w402 -> [_ w424]
                      tunnel: [w422 w426] -> w406
                      tunnel: w403 -> [w422 w425]
                      frame False {
                      }
                      frame True {
                        n129 = call <vilib>:"VIAn Remove Item.vi"("error in (no error)"=w425, "Item to Remove"=w424, "VI Analyzer Task in"=w428) -> ("error out"=w426:errorcluster, "VI Analyzer Task out"=w427:T2)  [unwired: 7 in]
                      }
                    }
                    n130 = Build Array(w402) -> (w401:path[])
                    n131 = Select(t=w401, s=w400, f=path[] []) -> (s? t:f=w399:path[])
                  }
                }
              }
              n132 = Array Size(array=w346) -> (size(s)=w345:i32)
              n133 = Format Into String(format string="Excluded %d Files" ("Text to Write"), w345) -> (resulting string=w337:string)  [unwired: 2 in, 1 out]
              n134 = call <vilib>:"Write Line.vi"("error in (no error)"=w341, "Text to Write"=w337, "CLI in"=w339) -> ("error out"=w340:errorcluster, "CLI out"=w338:refnum<class "CLI.lvclass">)  [unwired: 7 in]
            }
            frame True {
            }
          }
          n135 = in-place-cluster #3("Viancfg Path"=w323, "CLI"=w332, "VI Analyzer Task"=w329, "Excluded Folders"=w326) -> (w321:T11)
        }
      }
      frame "Run viancfg" {
        n136 = in-place {
          in-place-border: w436 -> [w446]
          in-place-border: [w460] -> w435
          in-place-border: [VI_Analyzer_State."Report Threshold"] -> w434
          n137 = in-place-cluster #4(w438) -> ("CLI"=w442:refnum<class "CLI.lvclass">, "VI Analyzer Task"=w445:T2)  [unwired: 1 out]
          n138 = call <vilib>:"VIAn Get Items.vi"("error in (no error)"=w446, "VI Analyzer Task in"=w445) -> ("error out"=w449:errorcluster, "Items"=w450:path[], "VI Analyzer Task out"=w444:T2)  [unwired: 7 in]
          n139 = for {
            tunnel: w450 -> [w471] mode=indexing
            tunnel: [w473] -> w451 mode=concatenating
            shift-right: [w472] -> w448
            shift-left: w449 -> [w468]
            n140 = File/Directory Info(path=w471, error in=w468) -> (path out=w469:path, directory=w470:bool, error out=w467:errorcluster)  [unwired: 4 out]
            n141 = case shown="True" w470 {
              tunnel: w469 -> [w476 w481]
              tunnel: [w475 w480] -> w473
              tunnel: w467 -> [w474 w479]
              tunnel: [w474 w478] -> w472
              frame False {
                n142 = Build Array(w476) -> (w475:path[])
              }
              frame True {
                n143 = call <vilib>:"Recursive File List.vi"("pattern"="*.vi", "error in (no error)"=w479, "Folder Path"=w481) -> ("error out"=w478:errorcluster, "All Files in Dir"=w480:path[])  [unwired: 4 in, 3 out]
              }
            }
          }
          "File Paths" <- w451
          n144 = Array Size(array=w451) -> (size(s)=w440:i32)
          "# VIs to Analyze" <- w440
          n145 = Format Into String(format string="Loaded %d files to analyze.", w440) -> (resulting string=w452:string)  [unwired: 2 in, 1 out]
          n146 = call <vilib>:"Write Line.vi"("error in (no error)"=w448, "Text to Write"=w452, "CLI in"=w442) -> ("error out"=w443:errorcluster, "CLI out"=w441:refnum<class "CLI.lvclass">)  [unwired: 7 in]
          n147 = call <vilib>:"Write Line.vi"("error in (no error)"=w443, "Text to Write"="Analyzing...", "CLI in"=w441) -> ("error out"=w458:errorcluster, "CLI out"=w465:refnum<class "CLI.lvclass">)  [unwired: 7 in]
          n148 = while {
            tunnel: w444 -> [w497]
            shift-right: [w495] -> w466
            shift-left: w465 -> [w496]
            shift-right: [w486] -> w457
            shift-left: w458 -> [w485]
            shift-right: [w483] -> _
            shift-left: -1.0 ("y") -> [w484]
            stop <- w491 stop-if-true
            n149 = call <vilib>:"VIAn Get Analysis Status.vi"("error in (no error)"=w485, "VI Analyzer Task in"=w497) -> ("error out"=w498:errorcluster, "VI in Analysis"=→"VI in Analysis":string, "Percent Complete"=w487:dbl)  [unwired: 6 in, 1 out]
            "% Complete" <- w487
            n150 = Greater Or Equal?(x=w487, y=99.0) -> (x >= y?=w489:bool)
            n151 = Or(x=w498, y=w489) -> (x .or. y?=w491:bool)
            n152 = Format Into String(format string="%.1f %% Complete", w487) -> (resulting string=w492:string)  [unwired: 2 in, 1 out]
            n153 = Quotient & Remainder(x=w487, y=5.0) -> (floor(x/y)=w483:dbl)  [unwired: 1 out]
            n154 = Not Equal?(x=w483, y=w484) -> (x != y?=w482:bool)
            n155 = case shown="True" w482 {
              tunnel: w496 -> [w500 w505]
              tunnel: [w500 w504] -> w495
              tunnel: w492 -> [_ w503]
              tunnel: w485 -> [w499 w502]
              tunnel: [w499 w501] -> w486
              frame False {
              }
              frame True {
                n156 = call <vilib>:"Write Line.vi"("error in (no error)"=w502, "Text to Write"=w503, "CLI in"=w505) -> ("error out"=w501:errorcluster, "CLI out"=w504:refnum<class "CLI.lvclass">)  [unwired: 7 in]
              }
            }
          }
          n157 = call <vilib>:"VIAn Run.vi"("Show Results Window?"="Show Results Window?", "error in (no error)"=w458, "VI Analyzer Task in"=w444) -> ("error out"=w456:errorcluster, "Analysis Results"=w459:T18, "VI Analyzer Task out"=w461:T2)  [unwired: 4 in, 2 out]
          n158 = Merge Errors(w456, w457) -> (w455:errorcluster)
          n159 = call <vilib>:"Write Line.vi"("error in (no error)"=w455, "Text to Write"="100% Complete", "CLI in"=w466) -> ("error out"=w460:errorcluster, "CLI out"=w462:refnum<class "CLI.lvclass">)  [unwired: 7 in]
          n160 = in-place-cluster #4("CLI"=w462, "VI Analyzer Task"=w461, "Analysis Results"=w459) -> (w437:T11)
        }
      }
      frame "Report Threshold" {
        n161 = in-place {
          in-place-border: w509 -> [w522]
          in-place-border: [w524] -> w508
          in-place-border: [VI_Analyzer_State."Report HTML"] -> w507
          in-place-border: w506 -> [w521]
          n162 = in-place-cluster #5(w506) -> ("CLI"=w525:refnum<class "CLI.lvclass">)  [unwired: 1 out]
          n163 = Unbundle By Name(w521) -> ("Analysis Results"=w520:T18, "Report Directory"=w517:path, "Working Directory"=w519:path, "Ranking Thresholds"=w518:T1, "Per VI Threshold"=w514:bool)
          n164 = call "Grade VIA Results.vi"("Grade Per Ranking? (T)"=w514, "Repo Root"=w519, "Error in"=w522, "Ranking Thresholds"=w518, "VIAResult"=w520) -> ("Error out"=w516:errorcluster, "Pass?"=w511:bool, "Individual VI Results"=w513:string, "VIA+ Results"=w512:string)  [unwired: 3 in]
          "Results" <- w512
          n165 = case shown="True" w514 {
            tunnel: w516 -> [w527 w532]
            tunnel: [w527 w531] -> w515
            tunnel: w517 -> [_ w530]
            tunnel: [_ w529] -> _
            tunnel: w513 -> [_ w528]
            frame False {
            }
            frame True {
              n166 = Build Path(base path=w530, name or relative path="IndividualVIRankings.csv") -> (appended path=w539:path)
              n167 = Open/Create/Replace File(file path (use dialog)=w539, error in=w532, operation (0:open)=T16."replace or create") -> (refnum out=w535:refnum<file>, error out=w536:errorcluster)  [unwired: 3 in, 1 out]
              n168 = Write to Text File(file (use dialog)=w535, text=w528, error in=w536) -> (refnum out=w533:refnum<file>, error out=w534:errorcluster)  [unwired: 1 in, 1 out]
              n169 = Close File(refnum=w533, error in=w534) -> (path=w529:path, error out=w531:errorcluster)
            }
          }
          n170 = call <vilib>:"Write Line.vi"("error in (no error)"=w515, "Text to Write"=w512, "CLI in"=w525) -> ("error out"=w524:errorcluster, "CLI out"=w526:refnum<class "CLI.lvclass">)  [unwired: 7 in]
          n171 = in-place-cluster #5("CLI"=w526, "Threshold Pass"=w511) -> (w510:T11)
        }
      }
      frame "Report HTML" {
        n172 = in-place {
          in-place-border: w543 -> [w546]
          in-place-border: [w552] -> w542
          in-place-border: [VI_Analyzer_State."Report RSL"] -> w541
          in-place-border: w540 -> [w550]
          n173 = in-place-cluster #6(w540) -> ("CLI"=w548:refnum<class "CLI.lvclass">)
          n174 = Unbundle By Name(w550) -> ("Analysis Results"=w549:T18, "Report Directory"=w547:path, "HTML Report"=w545:bool)
          n175 = case shown="True" w545 {
            tunnel: [w554 w569] -> w553
            tunnel: [w555 w568] -> w552
            tunnel: w549 -> [_ w565]
            tunnel: w548 -> [w554 w564]
            tunnel: w547 -> [_ w559]
            tunnel: w546 -> [w555 w558]
            frame False {
            }
            frame True {
              w571 = u16 1 items=["ASCII", "HTML", "RSL File"] ("Report Save Type (ASCII)")
              n176 = call <vilib>:"Create Directory Recursive.vi"("error in (no error)"=w558, "directory"=w559) -> ("error out"=w557:errorcluster, "directory copy"=w556:path)  [unwired: 3 in, 1 out]
              n177 = Get Date/Time In Seconds() -> (seconds since 1Jan1904=w561:timestamp)
              n178 = Format Into String(format string="VIA_Results_%<%y_%m_%d_%H_%M>T.html", w561) -> (resulting string=w560:string)  [unwired: 2 in, 1 out]
              n179 = Build Path(base path=w556, name or relative path=w560) -> (appended path=w563:path)
              n180 = Format Into String(format string="Reporting HTML \"%s\"" ("Text to Write"), w563) -> (resulting string=w566:string)  [unwired: 2 in, 1 out]
              n181 = call <vilib>:"Write Line.vi"("error in (no error)"=w557, "Text to Write"=w566, "CLI in"=w564) -> ("error out"=w570:errorcluster, "CLI out"=w569:refnum<class "CLI.lvclass">)  [unwired: 7 in]
              n182 = call <vilib>:"VIAn Easy Report.vi"("Overwrite Report?  (T)"=TRUE, "error in (no error)"=w570, "Report Save Type (ASCII)"=w571, "Analysis Results"=w565, "Report Save Path"=w563) -> ("error out"=w568:errorcluster)  [unwired: 6 in]
            }
          }
          n183 = in-place-cluster #6("CLI"=w553) -> (w544:T11)
        }
      }
      frame "Report RSL" {
        n184 = in-place {
          in-place-border: w576 -> [w579]
          in-place-border: [w585] -> w575
          in-place-border: [VI_Analyzer_State."Close"] -> w574
          in-place-border: w573 -> [w583]
          n185 = in-place-cluster #7(w573) -> ("CLI"=w581:refnum<class "CLI.lvclass">)
          n186 = Unbundle By Name(w583) -> ("Analysis Results"=w582:T18, "Report Directory"=w580:path, "RSL Report"=w578:bool)
          n187 = case shown="True" w578 {
            tunnel: [w587 w602] -> w586
            tunnel: [w588 w601] -> w585
            tunnel: w582 -> [_ w598]
            tunnel: w581 -> [w587 w597]
            tunnel: w580 -> [_ w596]
            tunnel: w579 -> [w588 w595]
            frame False {
            }
            frame True {
              w604 = u16 2 items=["ASCII", "HTML", "RSL File"] ("Report Save Type (ASCII)")
              n188 = call <vilib>:"Create Directory Recursive.vi"("error in (no error)"=w595, "directory"=w596) -> ("error out"=w594:errorcluster, "directory copy"=w593:path)  [unwired: 3 in, 1 out]
              n189 = Get Date/Time In Seconds() -> (seconds since 1Jan1904=w590:timestamp)
              n190 = Format Into String(format string="VIA_Results_%<%y_%m_%d_%H_%M>T.rsl", w590) -> (resulting string=w589:string)  [unwired: 2 in, 1 out]
              n191 = Build Path(base path=w593, name or relative path=w589) -> (appended path=w592:path)
              n192 = Format Into String(format string="Reporting RSL \"%s\"" ("Text to Write"), w592) -> (resulting string=w599:string)  [unwired: 2 in, 1 out]
              n193 = call <vilib>:"Write Line.vi"("error in (no error)"=w594, "Text to Write"=w599, "CLI in"=w597) -> ("error out"=w603:errorcluster, "CLI out"=w602:refnum<class "CLI.lvclass">)  [unwired: 7 in]
              n194 = call <vilib>:"VIAn Easy Report.vi"("Overwrite Report?  (T)"=TRUE, "error in (no error)"=w603, "Report Save Type (ASCII)"=w604, "Analysis Results"=w598, "Report Save Path"=w592) -> ("error out"=w601:errorcluster)  [unwired: 6 in]
            }
          }
          n195 = in-place-cluster #7("CLI"=w586) -> (w577:T11)
        }
      }
      frame "Close" {
        n196 = Unbundle By Name(w619) -> ("Threshold Pass"=w606:bool, "CLI"=w613:refnum<class "CLI.lvclass">, "VI Analyzer Task"=w617:T2)
        n197 = call <vilib>:"Write Line.vi"("Text to Write"="Exiting VI Analzyer", "CLI in"=w613) -> ("CLI out"=w612:refnum<class "CLI.lvclass">)  [unwired: 8 in, 1 out]
        n198 = call <vilib>:"VIAn Destroy Task.vi"("error in (no error)"=w618, "VI Analyzer Task in"=w617) -> ("error out"=w616:errorcluster)  [unwired: 9 in]
        n199 = Select(t=0, s=w606, f=1 ("No Error Code (0)")) -> (s? t:f=w608:i32)
        n200 = call <vilib>:"Exit With Error Cluster Code.vi"("error in (no error)"=w616, "No Error Code (0)"=w608, "CLI in"=w612) -> ("error out"=w615:errorcluster)  [unwired: 8 in]
      }
      frame "Help" {
        n201 = in-place {
          in-place-border: w623 -> [w630]
          in-place-border: [w629] -> w622
          n202 = in-place-cluster #8(w621) -> ("CLI"=w628:refnum<class "CLI.lvclass">)  [unwired: 1 out]
          n203 = call <vilib>:"Write Line.vi"("error in (no error)"=w630, "Text to Write"="-------optional arguments-------\n-viancfg <absolute or relative to working directory relative path to viancfg file. defaults to Default.viancfg included with app>\n-reportdir <absolute or relative to working directory relative path to report output directory. Defaults to workingdir/Reports>\n-included <comma seperated string of all folders within working directory to include. Recursive search. Defaults to settings within viancfg>\n-excluded <comma seperated string of all folders within working directory to exclude. Defaults to none>\n-high <High Threshold, default 100>\n-normal <Normal Threshold, default 100>\n-low <Low Threshold, default 100>\n-pervi <Flag to run thresholds against each VI instead of catagories>\n-html <Flag to generate html report>\n-rsl <Flag to generate rsl report>\n-help <Returns this help information>" ("string"), "CLI in"=w628) -> ("error out"=w629:errorcluster, "CLI out"=w627:refnum<class "CLI.lvclass">)  [unwired: 7 in]
          n204 = in-place-cluster #8("CLI"=w627, "Threshold Pass"=TRUE) -> (w620:T11)
        }
      }
    }
    n205 = Select(t=VI_Analyzer_State."Close", s=w9, f=w7) -> (s? t:f=w6:T12)
  }
  n206 = invoke class="VI" method="FP.Close"(error in=w1) -> ()  [unwired: 2 in, 3 out]
